vi "PrefDialog.vi"(8 "error in (no error)":errorcluster, 11 "MyPluginsBase in":refnum<class "NHRDCPowerModel.lvclass">) -> (0 "error out":errorcluster, 1 "Save As":bool, 2 "Changed":bool, 3 "MyPluginsBase out":refnum<class "NHRDCPowerModel.lvclass">)   [LabVIEW 2018, in "AcPwrPlugins.lvlib" / "NHRDCPowerModel.lvclass"]
doc: "This VI displays the prior instruments properties and allows a user to change the instrument properties and save these new set properties to the same location on disk or in a new location with a new name called \"Type\"."
uses:
  NHRDCPowerModel.lvclass
  F:/Program Files (x86)/National Instruments/LabVIEW 2018/user.lib/NIST/BaseClasses/BasePlugin_class/BasePlugin.lvclass
  F:/Projects/ICDAS/NistPluggableModules/AcPwr/AcPwrPlugins/AcPwrBaseClass/AcPwrBase.lvclass
  NHRDCPowerClass/TypeDefs/Device(s)Settings.ctl
  NHRDCPowerClass/TypeDefs/Modules.ctl
  NHRDCPowerClass/TypeDefs/Measurements.ctl
  AcPwrShared/Database Settings.ctl
  <userlib>/NIST/BaseClasses/BasePlugin_class/BasePlugin.lvclass/BasePlugin.ctl
  AcPwrBaseClass/AcPwrBase.lvclass/AcPwrBase.ctl
  <userlib>/NIST/BaseClasses/BasePlugin_class/Accessors/Read PluginIniFilePath.vi
  AcPwrBaseClass/Accessors/Read BaseConfig.vi
  AcPwrBaseClass/Accessors/Read BaseMeasurements.vi
  <userlib>/NIST/BaseClasses/BasePlugin_class/Accessors/Write PluginIniFilePath.vi
  <vilib>/Utility/config.llb/NI_LVConfig.lvlib
  AcPwrBaseClass/AcPwrBase.lvclass
  NHRDCPowerClass/NHRDCPower.lvclass
  AcPwrShared/AcPwrShared.lvlib
panel:
  in  "Database Settings":T1
  in  "btnSaveAs":bool
  in  "btnSave":bool
  in  "Measurement RefreshTime (ms)":u32
  in  "btnCancel":bool
  in  "Measurements":T2
  in  "Device(s)Settings":T3 {"Modules"."Regulation Gain (1=100%)" min=0.0 max=1.0; "Modules"."OutputSettings"."Wait on Value" items=["Voltage Greater Than Or Equal To", "Voltage Less Than Or Equal To", "Current Greater Than Or Equal To", "Current Less Than Or Equal To", "Power Greater Than Or Equal To", "Power Less Than Or Equal To"]; "Modules"."operating state (Off)" items=["Off", "Stand By", "Charge", "Discharge", "Battery Emulation"]}
  # "*Please ensure that Voltage and Current are selected as the 1st and 2nd Measurement variables, respectively, to correctly plot Voltage vs Current in the visualization VI."
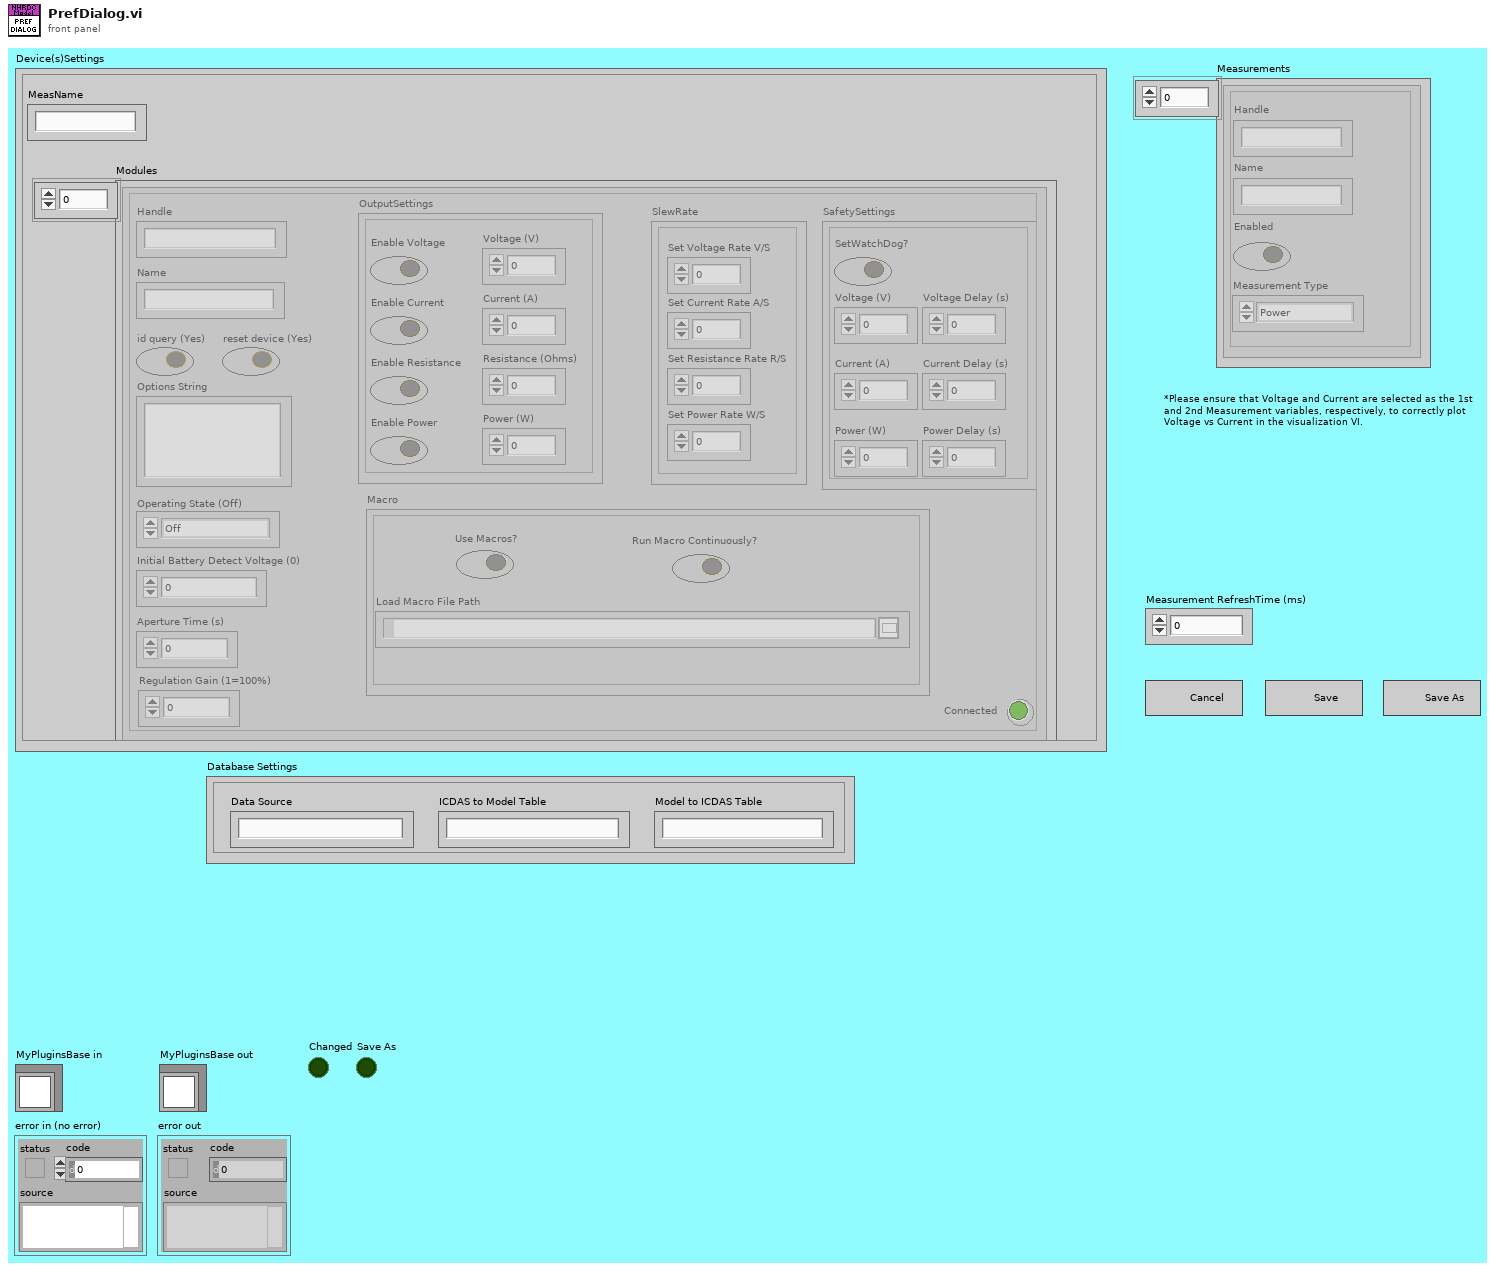
[diagram p1: front panel]
types:
  T1 = typedef "AcPwrShared.lvlib/Database Settings.ctl" = cluster{"Data Source":string, "ICDAS to Model Table":string, "Model to ICDAS Table":string}
  T2 = typedef "AcPwrPlugins.lvlib/NHRDCPower.lvclass/Measurements.ctl" = cluster{"Handle":string, "Name":string, "Enabled":bool, "Measurement Value":sgl, "Measurement Type":enum16{"Power", "Current", "Voltage"}}[]
  T3 = typedef "AcPwrPlugins.lvlib/NHRDCPower.lvclass/Device(s)Settings.ctl" = cluster{"MeasName":string, "Modules":T4}
  T4 = typedef "AcPwrPlugins.lvlib/NHRDCPower.lvclass/Modules.ctl" = cluster{"Handle":string, "Name":string, "id query (Yes)":bool, "reset device (Yes)":bool, "Connected":bool, "Initial Battery Detect Voltage (0)":dbl, "SafetySettings":cluster{"SetWatchDog?":bool, "Voltage (V)":dbl, "Current (A)":dbl, "Power (W)":dbl, "Voltage Delay (s)":dbl, "Current Delay (s)":dbl, "Power Delay (s)":dbl}, "Options String":string, "Aperture Time (s)":dbl, "operating state (Off)":i32, "OutputSettings":cluster{"Voltage (V)":dbl, "Current (A)":dbl, "Resistance (Ohms)":dbl, "Power (W)":dbl, "Enable Voltage":bool, "Enable Current":bool, "Enable Resistance":bool, "Enable Power":bool, "Macro After Step Delay  (s)":dbl, "Wait Value (V, A, W)":dbl, "Enable Wait":bool, "Wait on Value":i32}, "SlewRate":cluster{"Set Voltage Rate V/S":dbl, "Set Current Rate A/S":dbl, "Set Resistance Rate R/S":dbl, "Set Power Rate W/S":dbl}, "Macro":cluster{"Save Macro?":bool, "Load Macro From File?":bool, "Run Macro Continuously?":bool, "Use Macros?":bool, "Load Macro File Path":path, "Save Macro File Path":string}, "Regulation Gain (1=100%)":dbl, "UpdatingOntheFly":bool}[]
  T5 = enum8{"Enabled", "Disabled", "Disabled and Grayed Out"}
  T6 = enum32{"Invalid", "Default", "Floating", "Floating/Auto-Hide", "Modal"}
  T7 = cluster{"Device(s)Settings":T3, "Database Settings":T1}
  T8 = cluster{"Handle":string, "Name":string, "id query (Yes)":bool, "reset device (Yes)":bool, "Connected":bool, "Initial Battery Detect Voltage (0)":dbl, "SafetySettings":cluster{"SetWatchDog?":bool, "Voltage (V)":dbl, "Current (A)":dbl, "Power (W)":dbl, "Voltage Delay (s)":dbl, "Current Delay (s)":dbl, "Power Delay (s)":dbl}, "Options String":string, "Aperture Time (s)":dbl, "operating state (Off)":i32, "OutputSettings":cluster{"Voltage (V)":dbl, "Current (A)":dbl, "Resistance (Ohms)":dbl, "Power (W)":dbl, "Enable Voltage":bool, "Enable Current":bool, "Enable Resistance":bool, "Enable Power":bool, "Macro After Step Delay  (s)":dbl, "Wait Value (V, A, W)":dbl, "Enable Wait":bool, "Wait on Value":i32}, "SlewRate":cluster{"Set Voltage Rate V/S":dbl, "Set Current Rate A/S":dbl, "Set Resistance Rate R/S":dbl, "Set Power Rate W/S":dbl}, "Macro":cluster{"Save Macro?":bool, "Load Macro From File?":bool, "Run Macro Continuously?":bool, "Use Macros?":bool, "Load Macro File Path":path, "Save Macro File Path":string}, "Regulation Gain (1=100%)":dbl, "UpdatingOntheFly":bool}
  T9 = typedef "AcPwrPlugins.lvlib/AcPwrBase.lvclass/BaseConfig.ctl" = cluster{"Frequency":dbl, "FrequencyRange":dbl[], "Phases":T10[], "Name":string, "PluginConfigVariant":variant, "PluginMeasVariant":variant}
  T10 = typedef "AcPwrPlugins.lvlib/AcPwrBase.lvclass/Phase.ctl" = cluster{"Name":string, "Enabled":bool, "VoltageLevel":dbl, "Handle":string, "VoltageRange":dbl[], "Connected":bool, "CurrentLimit":dbl, "Waveform":string}
  T11 = typedef "AcPwrPlugins.lvlib/AcPwrBase.lvclass/BaseMeasurements.ctl" = cluster{"Handle":string, "Name":string, "Enabled":bool, "Measurement Value":dbl, "btnMeasFetch":bool, "Chroma Hold Peak Current Measurement":bool, "Chroma Measurement Type":T12, "Chroma Protection Status String":string, "NHRDC Fetch Method":i32, "NHRDC Fetch Time (s)":sgl, "NHRDC Measurement Type":i32, "NHRGridSim Measurement Type ":enum16{"Average Current", "Max Current", "Min Current", "Average Voltage", "Max Voltage", "Min Voltage", "Average True Power", "Max True Power", "Min True Power", "Average Apparent Power", "Max Apparent Power", "Min Apparent Power", "Power Factor", "Crest Factor"}, "NHRGridSim Phase ":i32, "PPS Measurement Type ":enum16{"Voltage RMS L-N", "Voltage RMS L-L", "Frequency", "Current RMS", "Current Peak", "Crest Factor", "Power Factor", "Power VA", "Real Power"}, "PPS Channel Name":enum16{"A", "B", "C"}}[]
  T12 = typedef "AcPwrPlugins.lvlib/ChromaAcLoad.lvclass/MeasurementType.ctl" = enum16{"Voltage (Vrms or V)", "Current (Arms or A)", "Power (W)", "Peak Voltage (V)", "Peak Current (A)", "Peak Power (W)", "Frequency (Hz)", "Resistance (Ohms)", "Voltage Overshoot (V)", "Positive Peak Current (A)", "Voltage Undershoot (V)", "Negative Peak Current (A)", "Apparent Power (VA)", "Reacitive Power (VAR)", "Voltage THD", "Power Factor", "Current's Crest Factor"}
  T13 = typedef "NI_LVConfig.lvlib/Config Data RefNum.ctl" = refnum<k1>
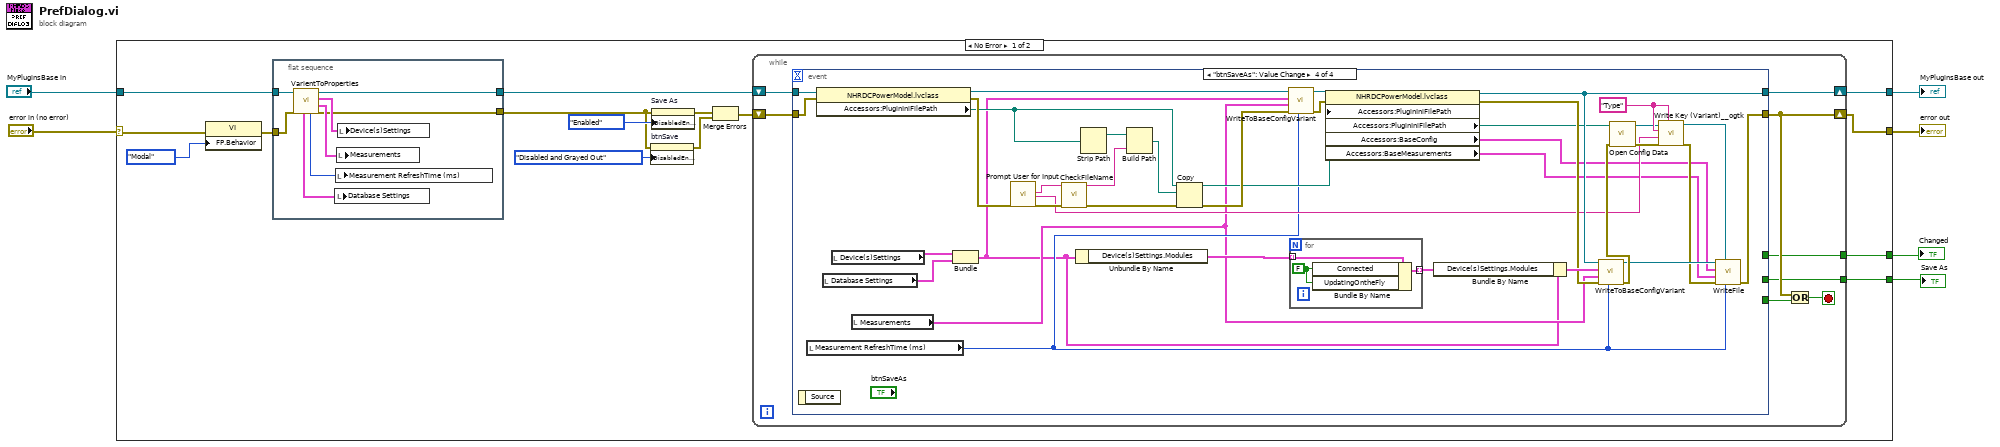
[diagram p0: block diagram]
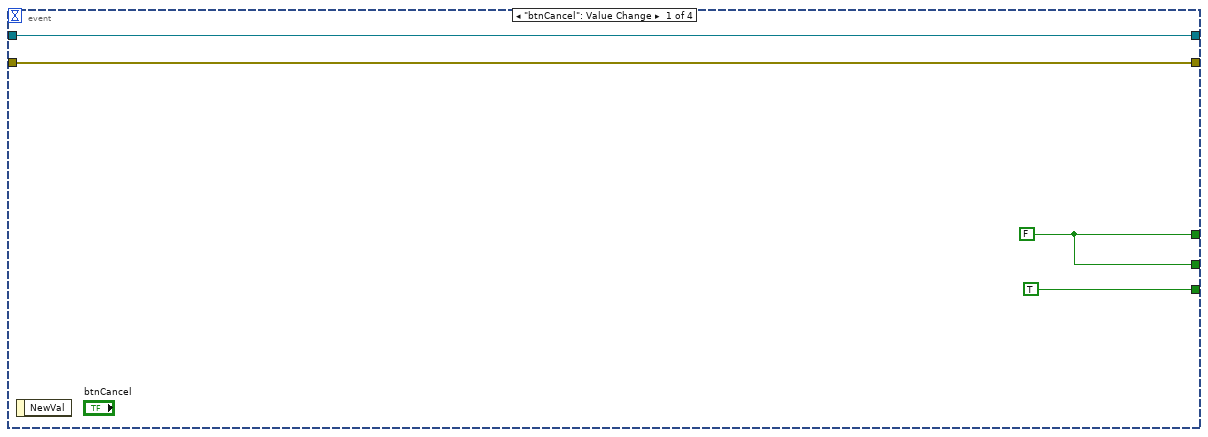
[diagram p2: hidden frame]
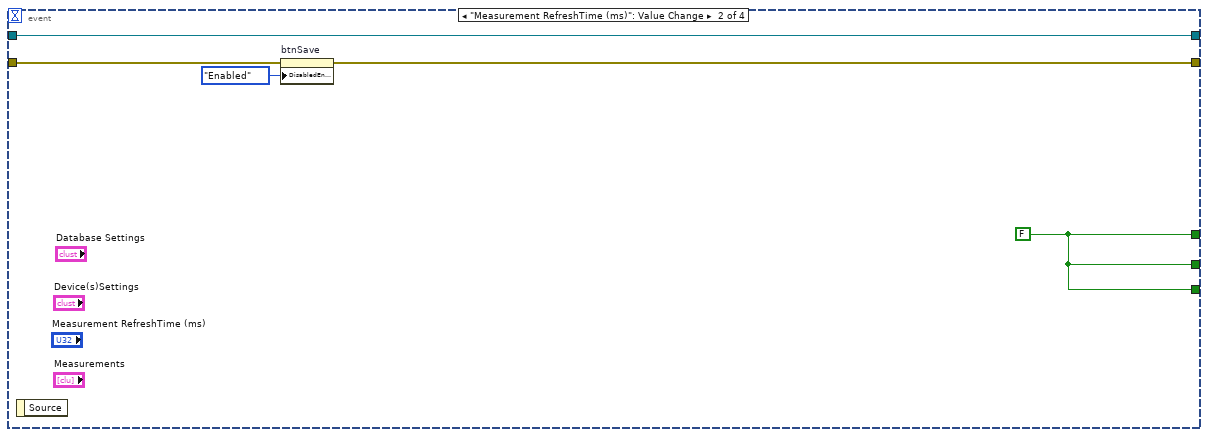
[diagram p3: hidden frame]
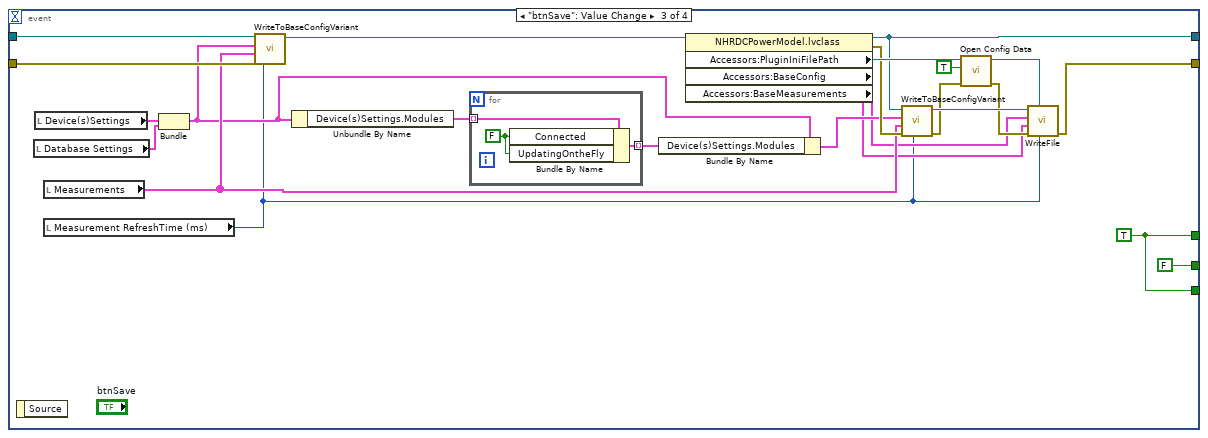
[diagram p4: hidden frame]
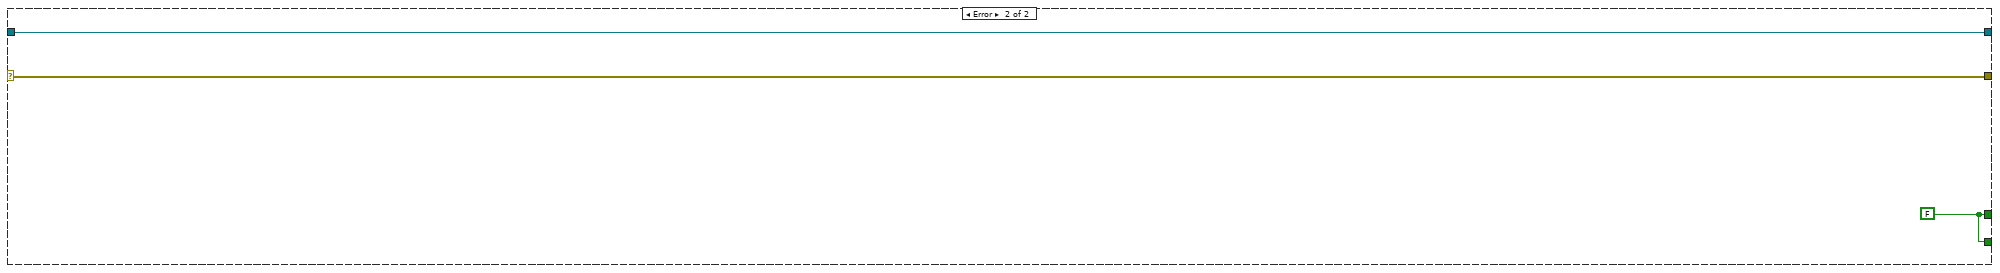
[diagram p5: hidden frame]
diagram:
  n1 = case shown="No Error" "error in (no error)" {
    selector: "error in (no error)" -> [w20 w115]
    tunnel: "MyPluginsBase in" -> [w19 w116]
    tunnel: [w10 w116] -> w4
    tunnel: [w9 w115] -> w3
    tunnel: [w8 w114] -> w2
    tunnel: [w7 w114] -> w1
    frame No Error {
      n2 = property class="VI"(error in=w20, "FP.Behavior"=T6."Modal" ("Front Panel Window:Behavior")) -> (error out=w18:errorcluster)  [unwired: 1 in, 1 out]
      n3 = flat-sequence {
        tunnel: w19 -> [w113]
        tunnel: w18 -> [w112]
        tunnel: [w108] -> w12
        tunnel: [w107] -> w16
        frame #0 {
          n4 = call "VarientToProperties.vi"("error in (no error)"=w112, "AcPwrPlugins.lvlib:NHRDCModel.lvclass"=w113) -> ("error out"=w107:errorcluster, "Measurements"=w110:T2, "Device(s)Settings"=w111:T3, "AcPwrPlugins.lvlib:NHRDCModel.lvclass"=w108:refnum<class "NHRDCPowerModel.lvclass">, "Measurement Refresh Time (ms)"=w109:u32, "Database Settings"=w106:T1)  [unwired: 4 in]
          n5 = local write "Database Settings"(w106) -> ()
          n6 = local write "Measurement RefreshTime (ms)"(w109) -> ()
          n7 = local write "Measurements"(w110) -> ()
          n8 = local write "Device(s)Settings"(w111) -> ()
        }
      }
      n9 = property on="btnSave" class="Bool"(error in=w16, "DisabledEnum"=T5."Disabled and Grayed Out" ("Disabled")) -> (error out=w13:errorcluster)  [unwired: 1 in, 1 out]
      n10 = property on="Save As" class="Bool (strict)"(error in=w16, "DisabledEnum"=T5."Enabled" ("Disabled")) -> (error out=w14:errorcluster)  [unwired: 1 in, 1 out]
      n11 = Merge Errors(w14, w13) -> (w11:errorcluster)
      n12 = while {
        shift-right: [w24] -> w10
        shift-left: w12 -> [w29]
        shift-right: [w25] -> w9
        shift-left: w11 -> [w28]
        tunnel: [w23] -> w8
        tunnel: [w22] -> w7
        stop <- w26 stop-if-true
        n13 = event shown="[3] \"btnSaveAs\": Value Change" {
          selector: _ -> [_ _ _ _]
          dyn-events: _ -> [_ _ _ _]
          timeout: _ -> [_ _ _ _]
          tunnel: w29 -> [w30 w34 w62 w102]
          tunnel: w28 -> [w33 w38 w61 w101]
          tunnel: [w33 w36 w45 w73] -> w25
          tunnel: [TRUE w35 w43 _] -> w27
          tunnel: [w31 w35 w43 _] -> w23
          tunnel: [w31 w35 FALSE _] -> w22
          tunnel: [w30 w34 w55 w86] -> w24
          event "btnCancel": Value Change {
            w31 = FALSE
            n14 = event-data() -> ()  [unwired: 1 in, 1 out]
          }
          event "Measurement RefreshTime (ms)": Value Change {
            w35 = FALSE
            n15 = event-data() -> ()  [unwired: 1 in, 1 out]
            n16 = property on="btnSave" class="Bool"(error in=w38, "DisabledEnum"=T5."Enabled" ("Disabled")) -> (error out=w36:errorcluster)  [unwired: 1 in, 1 out]
          }
          event "btnSave": Value Change {
            w43 = TRUE
            n17 = event-data() -> ()  [unwired: 1 in, 1 out]
            n18 = local read "Database Settings"() -> (w42:T1)
            n19 = local read "Device(s)Settings"() -> (w41:T3)
            n20 = local read "Measurements"() -> (w52:T2)
            n21 = local read "Measurement RefreshTime (ms)"() -> (w39:u32)
            n22 = Bundle("Device(s)Settings"=w41, "Database Settings"=w42) -> (w40:T7)  [unwired: 1 in]
            n23 = call-dynamic "WriteToBaseConfigVariant.vi"("Measurement Refresh Time (ms)"=w39, "error in (no error)"=w61, "Meas"=w52, "Config"=w40, "NHRDCModel in"=w62) -> ("NHRDCModel out"=w58:refnum<class "NHRDCPowerModel.lvclass">)  [unwired: 5 in, 1 out]
            n24 = Unbundle By Name(w40) -> ("Device(s)Settings.Modules"=w60:T4)
            n25 = for {
              tunnel: w60 -> [w65] mode=indexing
              tunnel: [w63] -> w59 mode=indexing
              w64 = FALSE ("Connected")
              n26 = Bundle By Name(cluster=w65, "Connected"=w64, "UpdatingOntheFly"=w64) -> (w63:T8)
            }
            n27 = Bundle By Name(cluster=w40, "Device(s)Settings.Modules"=w59) -> (w53:T7)
            n28 = property class="NHRDCPowerModel.lvclass"(reference=w58) -> (reference out=w55:refnum<class "NHRDCPowerModel.lvclass">, error out=w54:errorcluster, "Accessors:PluginIniFilePath"=w57:path, "Accessors:BaseConfig"=w47:T9, "Accessors:BaseMeasurements"=w46:T11)  [unwired: 1 in]
            n29 = call-dynamic "WriteToBaseConfigVariant.vi"("Measurement Refresh Time (ms)"=w39, "error in (no error)"=w54, "Meas"=w52, "Config"=w53, "NHRDCModel in"=w55) -> ("error out"=w50:errorcluster, "NHRDCModel out"=w51:refnum<class "NHRDCPowerModel.lvclass">)  [unwired: 5 in]
            n30 = call <vilib>:"Open Config Data.vi"("error in (no error)"=w50, "create file if necessary (T)"=TRUE, "configuration file path"=w57) -> ("error out"=w49:errorcluster, "refnum"=w48:T13)  [unwired: 6 in, 1 out]
            n31 = call-dynamic "WriteFile.vi"("RefreshTime"=w39, "Refnum in"=w48, "error in (no error)"=w49, "BaseMeasurements"=w46, "BaseConfiguration"=w47, "NHRDCModel in"=w51) -> ("error out"=w45:errorcluster)  [unwired: 4 in, 1 out]
          }
          event "btnSaveAs": Value Change {
            w82 = "Type" ("section")
            n32 = event-data() -> ()  [unwired: 1 in, 1 out]
            n33 = local read "Measurement RefreshTime (ms)"() -> (w70:u32)
            n34 = property class="NHRDCPowerModel.lvclass"(reference=w102, error in=w101) -> (reference out=w93:refnum<class "NHRDCPowerModel.lvclass">, error out=w100:errorcluster, "Accessors:PluginIniFilePath"=w96:path)
            n35 = local read "Database Settings"() -> (w68:T1)
            n36 = local read "Device(s)Settings"() -> (w69:T3)
            n37 = local read "Measurements"() -> (w67:T2)
            n38 = Bundle("Device(s)Settings"=w69, "Database Settings"=w68) -> (w66:T7)  [unwired: 1 in]
            n39 = call "Prompt User for Input"("error in (no error)"=w100) -> ("File Name"=w78:string, "PluginType"=w77:string, "error out"=w99:errorcluster)  [unwired: 15 in, 1 out]
            n40 = call "CheckFileName.vi"("Error In"=w99, "File Name in"=w78) -> ("Error Out"=w94:errorcluster, "File Name out"=w97:string)  [unwired: 8 in]
            n41 = Unbundle By Name(w66) -> ("Device(s)Settings.Modules"=w88:T4)
            n42 = Strip Path(path=w96) -> (stripped path=w98:path)  [unwired: 1 out]
            n43 = Build Path(base path=w98, name or relative path=w97) -> (appended path=w95:path)
            n44 = Copy(8:w94, 10:w95, 11:w96) -> (0:w92:errorcluster, 3:w89:path)  [unwired: 2 in, 1 out]
            n45 = call-dynamic "WriteToBaseConfigVariant.vi"("Measurement Refresh Time (ms)"=w70, "error in (no error)"=w92, "Meas"=w67, "Config"=w66, "NHRDCModel in"=w93) -> ("error out"=w90:errorcluster, "NHRDCModel out"=w91:refnum<class "NHRDCPowerModel.lvclass">)  [unwired: 5 in]
            n46 = for {
              tunnel: w88 -> [w105] mode=indexing
              tunnel: [w104] -> w87 mode=indexing
              w103 = FALSE ("Connected")
              n47 = Bundle By Name(cluster=w105, "Connected"=w103, "UpdatingOntheFly"=w103) -> (w104:T8)
            }
            n48 = property class="NHRDCPowerModel.lvclass"(reference=w91, error in=w90, "Accessors:PluginIniFilePath"=w89) -> (reference out=w86:refnum<class "NHRDCPowerModel.lvclass">, error out=w84:errorcluster, "Accessors:PluginIniFilePath"=w83:path, "Accessors:BaseConfig"=w72:T9, "Accessors:BaseMeasurements"=w71:T11)
            n49 = Bundle By Name(cluster=w66, "Device(s)Settings.Modules"=w87) -> (w85:T7)
            n50 = call-dynamic "WriteToBaseConfigVariant.vi"("Measurement Refresh Time (ms)"=w70, "error in (no error)"=w84, "Meas"=w67, "Config"=w85, "NHRDCModel in"=w86) -> ("error out"=w79:errorcluster, "NHRDCModel out"=w76:refnum<class "NHRDCPowerModel.lvclass">)  [unwired: 5 in]
            n51 = call <vilib>:"Open Config Data.vi"("error in (no error)"=w79, "configuration file path"=w83) -> ("error out"=w80:errorcluster, "refnum"=w81:T13)  [unwired: 7 in, 1 out]
            n52 = call <userlib>:"Write Key (Variant)__ogtk.vi"("section"=w82, "error in (no error)"=w80, "key-value"=w77, "key (optional)"=w82, "refnum"=w81) -> ("error out"=w75:errorcluster, "refnum out"=w74:T13)  [unwired: 5 in]
            n53 = call-dynamic "WriteFile.vi"("RefreshTime"=w70, "Refnum in"=w74, "error in (no error)"=w75, "BaseMeasurements"=w71, "BaseConfiguration"=w72, "NHRDCModel in"=w76) -> ("error out"=w73:errorcluster)  [unwired: 4 in, 1 out]
          }
        }
        n54 = Or(x=w25, y=w27) -> (x .or. y?=w26:bool)
      }
    }
    frame Error {
      w114 = FALSE
    }
  }
  "error out" <- w3
  "MyPluginsBase out" <- w4
  "Save As" <- w1
  "Changed" <- w2
